vi "StageMoveDone.vi"(8 "error in (no error)":errorcluster, 10 "Positions":T1={"CH1 Pos"=0.0, "CH2 Pos"=0.0, "CH3 Pos"=0.0, "CH4 Pos"=0.0, "Home?"=TRUE}, 11 "TranslationStageUI.lvclass":refnum<class "TranslationStageUI.lvclass">) -> (0 "error out":errorcluster, 3 "TranslationStageUI.lvclass":refnum<class "TranslationStageUI.lvclass">)   [LabVIEW 2023, in "TranslationStage Library.lvlib" / "TranslationStage_UI.lvlib" / "TranslationStageUI.lvclass"]
uses:
  TranslationStageUI.lvclass
  StageMoveDone_For_UI.ctl
  TranslationStageUI.lvclass/TranslationStageUI.ctl
  typedefs/typedefs.lvlib
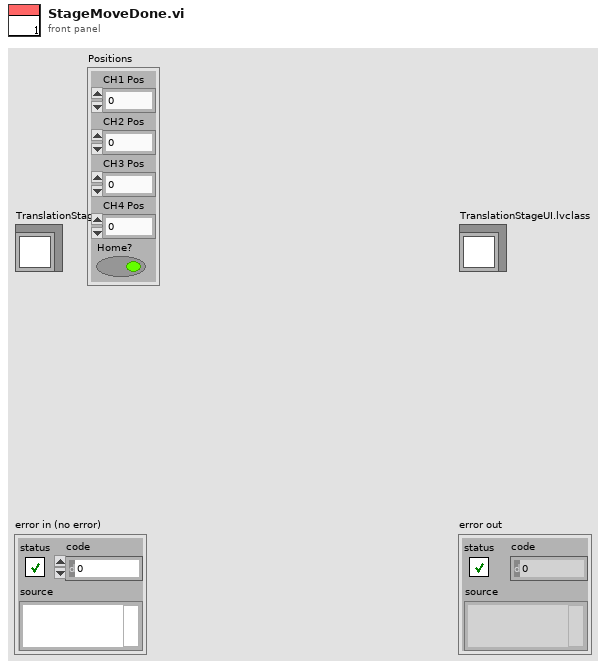
[diagram p1: front panel]
types:
  T1 = typedef "typedefs.lvlib/StageMoveDone_For_UI.ctl" = cluster{"CH1 Pos":sgl, "CH2 Pos":dbl, "CH3 Pos":dbl, "CH4 Pos":dbl, "Home?":bool}
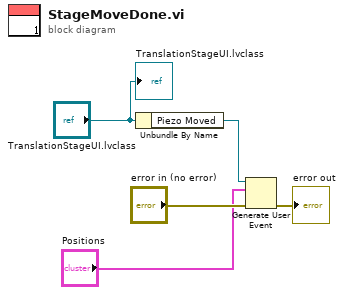
[diagram p0: block diagram]
diagram:
  n1 = Unbundle By Name("TranslationStageUI.lvclass") -> ("Piezo Moved"=w4:refnum<user-event>)
  n2 = Generate User Event(user event=w4, event data cluster="Positions", error in="error in (no error)") -> (error out=→"error out":errorcluster)  [unwired: 1 in, 1 out]
  "TranslationStageUI.lvclass" <- "TranslationStageUI.lvclass"
